vi "Calibraiton_Procedure.vi"(1 "timeout (ms)":i32=-1, 4 "error in":errorcluster, 5 "num_of_samples":i32, 6 "waveform_type":string, 7 "gRPC ID in":T2) -> (0 "error out":errorcluster, 2 "Response Data":T1, 3 "gRPC ID out":T2)   [LabVIEW 2024]
uses:
  FlexSDR_gRPC_client.lvlib
  RPC Messages/rfcontrol_RFDC.ctl
  RPC Messages/rfcontrol_RFDCSendWaveformRequest.ctl
  RPC Messages/rfcontrol_SetRFDCBackgroundCalibrationStateRequest.ctl
  RPC Messages/rfcontrol_RFDCCaptureWaveformRequest.ctl
  <vilib>/gRPC/LabVIEW gRPC Library/Shared/grpcId.ctl
  <vilib>/gRPC/LabVIEW gRPC Library/grpc-lvsupport-release.lvlib
  RPC Messages/rfcontrol_RFDCCaptureWaveformResponse.ctl
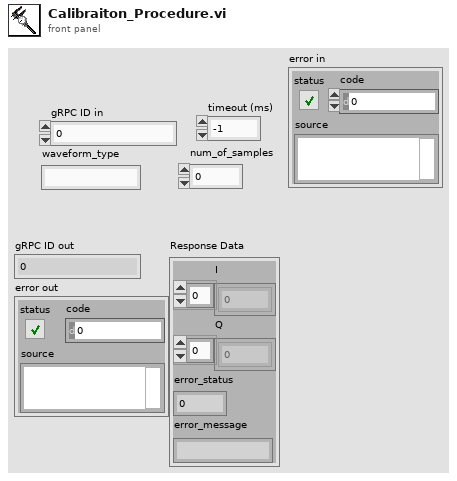
[diagram p1: front panel]
types:
  T1 = typedef "FlexSDR_gRPC_client.lvlib/rfcontrol_RFDCCaptureWaveformResponse.ctl" = cluster{"I":dbl[], "Q":dbl[], "error_status":i32, "error_message":string}
  T2 = typedef "grpc-lvsupport-release.lvlib/grpcId.ctl" = u64
  T3 = typedef "FlexSDR_gRPC_client.lvlib/rfcontrol_SetRFDCBackgroundCalibrationStateRequest.ctl" = cluster{"device_id":string, "rfdc":T4, "is_frozen":bool, "error_queue_populate":bool}
  T4 = typedef "FlexSDR_gRPC_client.lvlib/rfcontrol_RFDC.ctl" = enum32{"TX1", "TX2", "TX3", "TX4", "TX5", "TX6", "TX7", "TX8", "RX1", "RX2", "RX3", "RX4", "RX5", "RX6", "RX7", "RX8", "WRX1", "WRX2"}
  T5 = typedef "FlexSDR_gRPC_client.lvlib/rfcontrol_RFDCCaptureWaveformRequest.ctl" = cluster{"device_id":string, "rfdc":T4, "num_of_samples":i32, "error_queue_populate":bool}
  T6 = typedef "FlexSDR_gRPC_client.lvlib/rfcontrol_RFDCSendWaveformRequest.ctl" = cluster{"device_id":string, "rfdc":T4, "waveform_type":string, "error_queue_populate":bool}
  T7 = typedef "FlexSDR_gRPC_client.lvlib/rfcontrol_SetRFDCBackgroundCalibrationStateResponse.ctl" = cluster{"is_frozen":bool, "error_status":i32, "error_message":string}
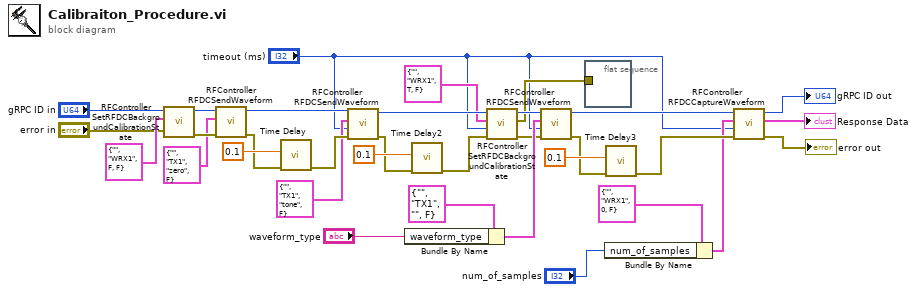
[diagram p0: block diagram]
diagram:
  n1 = call "RFController SetRFDCBackgroundCalibrationState.vi"("error in"="error in", "Request Data"=T3 {"device_id"="", "rfdc"=enum."WRX1", "is_frozen"=FALSE, "error_queue_populate"=FALSE}, "gRPC ID"="gRPC ID in") -> ("error out"=w32:errorcluster, "gRPC ID out"=w31:T2)  [unwired: 6 in, 1 out]
  n2 = call "RFController RFDCSendWaveform.vi"("error in"=w32, "Request Data"=T6 {"device_id"="", "rfdc"=enum."TX1", "waveform_type"="zero", "error_queue_populate"=FALSE}, "gRPC ID"=w31) -> ("error out"=w28:errorcluster, "gRPC ID out"=w27:T2)  [unwired: 6 in, 1 out]
  n3 = call "Time Delay"("error in (no error)"=w28, "Delay Time (s)"=0.1) -> ("error out"=w26:errorcluster)  [unwired: 9 in]
  n4 = call "RFController RFDCSendWaveform.vi"("error in"=w26, "timeout (ms)"="timeout (ms)", "Request Data"=T6 {"device_id"="", "rfdc"=enum."TX1", "waveform_type"="tone", "error_queue_populate"=FALSE}, "gRPC ID"=w27) -> ("error out"=w23:errorcluster, "gRPC ID out"=w14:T2)  [unwired: 5 in, 1 out]
  n5 = Bundle By Name(cluster=T6 {"device_id"="", "rfdc"=enum."TX1", "waveform_type"="", "error_queue_populate"=FALSE} ("Request Data"), "waveform_type"="waveform_type") -> (w21:T6)
  n6 = call "Time Delay2"("error in (no error)"=w23, "Delay Time (s)"=0.1) -> ("error out"=w13:errorcluster)  [unwired: 9 in]
  n7 = call "RFController SetRFDCBackgroundCalibrationState.vi"("error in"=w13, "timeout (ms)"="timeout (ms)", "Request Data"=T3 {"device_id"="", "rfdc"=enum."WRX1", "is_frozen"=TRUE, "error_queue_populate"=FALSE}, "gRPC ID"=w14) -> ("error out"=w12:errorcluster, "Response Data"=w9:T7, "gRPC ID out"=w11:T2)  [unwired: 5 in]
  n8 = call "RFController RFDCSendWaveform.vi"("error in"=w12, "timeout (ms)"="timeout (ms)", "Request Data"=w21, "gRPC ID"=w11) -> ("error out"=w19:errorcluster, "gRPC ID out"=w17:T2)  [unwired: 5 in, 1 out]
  n9 = flat-sequence {
    tunnel: w9 -> [_]
    frame #0 {
    }
  }
  n10 = Bundle By Name(cluster=T5 {"device_id"="", "rfdc"=enum."WRX1", "num_of_samples"=0, "error_queue_populate"=FALSE} ("Request Data"), "num_of_samples"="num_of_samples") -> (w15:T5)
  n11 = call "Time Delay3"("error in (no error)"=w19, "Delay Time (s)"=0.1) -> ("error out"=w18:errorcluster)  [unwired: 9 in]
  n12 = call "RFController RFDCCaptureWaveform.vi"("error in"=w18, "timeout (ms)"="timeout (ms)", "Request Data"=w15, "gRPC ID"=w17) -> ("error out"=→"error out":errorcluster, "Response Data"=→"Response Data":T1, "gRPC ID out"=→"gRPC ID out":T2)  [unwired: 5 in]
